vi "Set A Bit U16.vi"(9 "Input":u16 format="%08x", 10 "B":bool, 11 "Bit Number":u16) -> (3 "Output":u16 format="%08x")   [LabVIEW 2020]
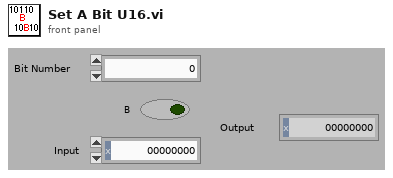
[diagram p1: front panel]
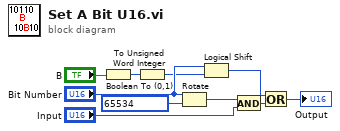
[diagram p0: block diagram]
diagram:
  n1 = Boolean To (0,1)(Boolean="B") -> (0, 1=w6:i16)
  n2 = To Unsigned Word Integer(number=w6) -> (unsigned 16bit integer=w2:u16)
  n3 = Rotate(1:u16 65534 ("x"), 2:"Bit Number") -> (0:w1:u16)
  n4 = Logical Shift(y="Bit Number", x=w2) -> (x << y=w3:u16)
  n5 = And(x=w1, y="Input") -> (x .and. y?=w8:u16)
  n6 = Or(x=w3, y=w8) -> (x .or. y?=→"Output":u16)
